vi "LV10_6.vi"() -> ()   [LabVIEW 2014]
uses:
  <vilib>/picture/picture.llb/Draw 8-Bit Pixmap.vi
panel:
  in  "Noise level":dbl(slide) scale=0.0..0.2
  out "Noisy image":picture
  out "Compression ratio":dbl
  in  "Threshold":dbl(slide) scale=0.01..1.0
  out "D3 wavelet transform":picture
  out "Original image":picture
  in  "Stop Button":bool
  out "Reconstructed image":picture
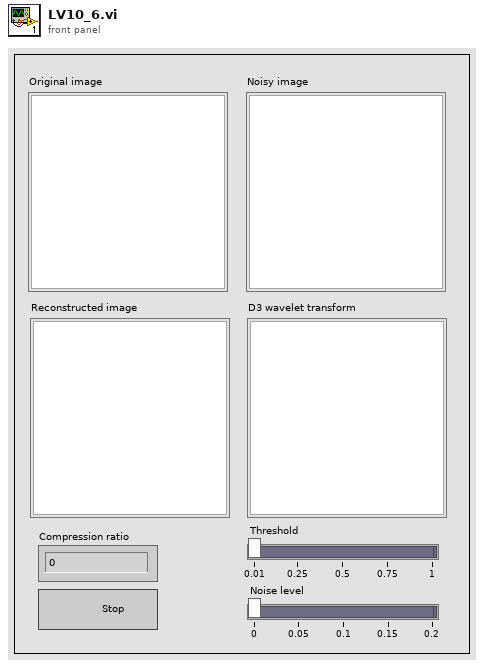
[diagram p1: front panel]
types:
  T1 = typedef "imagedata.ctl" = cluster{"image type":i32, "image depth":i32, "image":u8[], "mask":u8[], "colors":u32[], "Rectangle":cluster{"left":i16, "top":i16, "right":i16, "bottom":i16}}
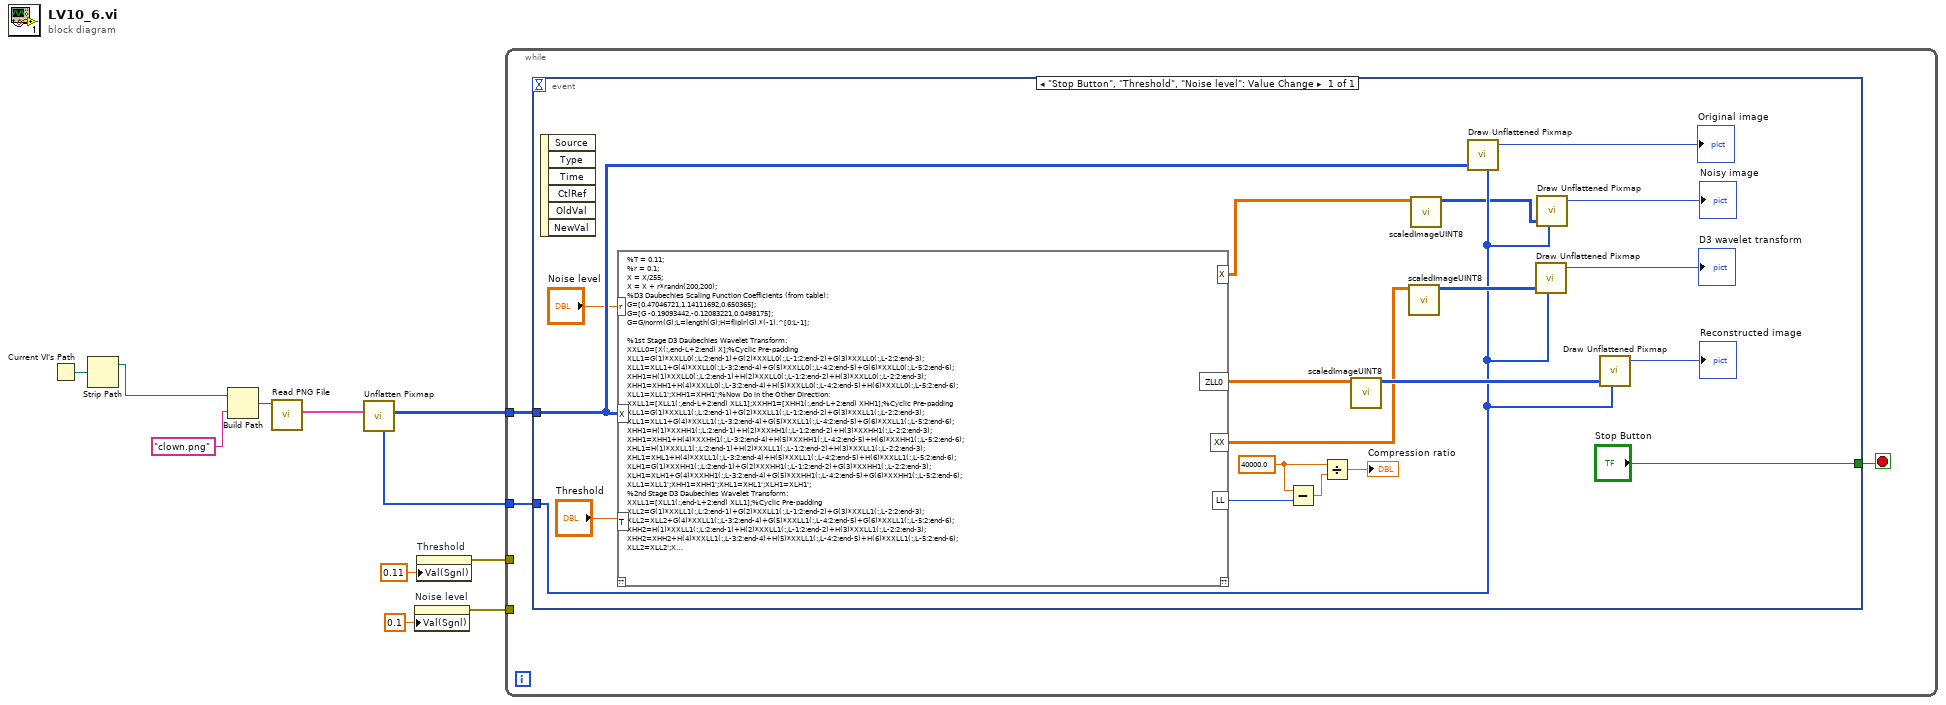
[diagram p0: block diagram]
diagram:
  n1 = Current VI's Path() -> (path=w11:path)
  n2 = Strip Path(path=w11) -> (stripped path=w1:path)  [unwired: 1 out]
  n3 = Build Path(base path=w1, name or relative path="clown.png") -> (appended path=w8:path)
  n4 = call <vilib>:"Read PNG File.vi"("path to PNG file"=w8) -> ("image data"=w7:T1)  [unwired: 8 in, 2 out]
  n5 = call <vilib>:"Unflatten Pixmap.vi"("image data"=w7) -> ("8-bit pixmap"=w9:u8[][], "colors"=w6:u32[])  [unwired: 4 in, 5 out]
  n6 = property on="Noise level" class="Slide (strict)"("Val(Sgnl)"=0.1 ("Value (Signaling)")) -> (error out=w3:errorcluster)  [unwired: 2 in, 1 out]
  n7 = property on="Threshold" class="Slide (strict)"("Val(Sgnl)"=0.11 ("Value (Signaling)")) -> (error out=w5:errorcluster)  [unwired: 2 in, 1 out]
  n8 = while {
    tunnel: w9 -> [w13]
    tunnel: w6 -> [w12]
    tunnel: w5 -> [_]
    tunnel: w3 -> [_]
    stop <- w14 stop-if-true
    n9 = event shown="[0] \"Stop Button\", \"Threshold\", \"Noise level\": Value Change" {
      selector: _ -> [_]
      dyn-events: _ -> [_]
      timeout: _ -> [_]
      tunnel: ["Stop Button"] -> w14
      tunnel: w13 -> [w30]
      tunnel: w12 -> [w17]
      event "Stop Button", "Threshold", "Noise level": Value Change {
        w24 = 40000.0 ("x")
        n10 = event-data() -> ()  [unwired: 1 in, 6 out]
        n11 = mathscript code="%T = 0.11;\n%r = 0.1;\nX = X/255;\nX = X + r*randn(200,200);\n%D3 Daubechies Scaling Function Coefficients (from table):\nG=[0.47046721,1.14111692,0.650365];\nG=[G -0.19093442,-0.12083221,0.0498175];\nG=G/norm(G);L=length(G);H=fliplr(G).*(-1).^[0:L-1];\n\n%1st Stage D3 Daubechies Wavelet Transform:\nXXLL0=[X(:,end-L+2:end) X];%Cyclic Pre-padding\nXLL1=G(1)*XXLL0(:,L:2:end-1)+G(2)*XXLL0(:,L-1:2:end-2)+G(3)*XXLL0(:,L-2:2:end-3);\nXLL1=XLL1+G(4)*XXLL0(:,L-3:2:end-4)+G(5)*XXLL0(:,L-4:2:end-5)+G(6)*XXLL0(:,L-5:2:end-6);\nXHH1=H(1)*XXLL0(:,L:2:end-1)+H(2)*XXLL0(:,L-1:2:end-2)+H(3)*XXLL0(:,L-2:2:end-3);\nXHH1=XHH1+H(4)*XXLL0(:,L-3:2:end-4)+H(5)*XXLL0(:,L-4:2:end-5)+H(6)*XXLL0(:,L-5:2:end-6);\nXLL1=XLL1';XHH1=XHH1';%Now Do in the Other Direction:\nXXLL1=[XLL1(:,end-L+2:end) XLL1];XXHH1=[XHH1(:,end-L+2:end) XHH1];%Cyclic Pre-padding\nXLL1=G(1)*XXLL1(:,L:2:end-1)+G(2)*XXLL1(:,L-1:2:end-2)+G(3)*XXLL1(:,L-2:2:end-3);\nXLL1=XLL1+G(4)*XXLL1(:,L-3:2:end-4)+G(5)*XXLL1(:,L-4:2:end-5)+G(6)*XXLL1(:,L-5:2:end-6);\nXHH1=H(1)*XXHH1(:,L:2:end-1)+H(2)*XXHH1(:,L-1:2:end-2)+H(3)*XXHH1(:,L-2:2:end-3);\nXHH1=XHH1+H(4)*XXHH1(:,L-3:2:end-4)+H(5)*XXHH1(:,L-4:2:end-5)+H(6)*XXHH1(:,L-5:2:end-6);\nXHL1=H(1)*XXLL1(:,L:2:end-1)+H(2)*XXLL1(:,L-1:2:end-2)+H(3)*XXLL1(:,L-2:2:end-3);\nXHL1=XHL1+H(4)*XXLL1(:,L-3:2:end-4)+H(5)*XXLL1(:,L-4:2:end-5)+H(6)*XXLL1(:,L-5:2:end-6);\nXLH1=G(1)*XXHH1(:,L:2:end-1)+G(2)*XXHH1(:,L-1:2:end-2)+G(3)*XXHH1(:,L-2:2:end-3);\nXLH1=XLH1+G(4)*XXHH1(:,L-3:2:end-4)+G(5)*XXHH1(:,L-4:2:end-5)+G(6)*XXHH1(:,L-5:2:end-6);\nXLL1=XLL1';XHH1=XHH1';XHL1=XHL1';XLH1=XLH1';\n%2nd Stage D3 Daubechies Wavelet Transform:\nXXLL1=[XLL1(:,end-L+2:end) XLL1];%Cyclic Pre-padding\nXLL2=G(1)*XXLL1(:,L:2:end-1)+G(2)*XXLL1(:,L-1:2:end-2)+G(3)*XXLL1(:,L-2:2:end-3);\nXLL2=XLL2+G(4)*XXLL1(:,L-3:2:end-4)+G(5)*XXLL1(:,L-4:2:end-5)+G(6)*XXLL1(:,L-5:2:end-6);\nXHH2=H(1)*XXLL1(:,L:2:end-1)+H(2)*XXLL1(:,L-1:2:end-2)+H(3)*XXLL1(:,L-2:2:end-3);\nXHH2=XHH2+H(4)*XXLL1(:,L-3:2:end-4)+H(5)*XXLL1(:,L-4:2:end-5)+H(6)*XXLL1(:,L-5:2:end-6);\nXLL2=XLL2';XHH2=XHH2';%Now Do in the Other Direction:\nXXLL2=[XLL2(:,end-L+2:end) XLL2];XXHH2=[XHH2(:,end-L+2:end) XHH2];%Cyclic Pre-padding\nXLL2=G(1)*XXLL2(:,L:2:end-1)+G(2)*XXLL2(:,L-1:2:end-2)+G(3)*XXLL2(:,L-2:2:end-3);\nXLL2=XLL2+G(4)*XXLL2(:,L-3:2:end-4)+G(5)*XXLL2(:,L-4:2:end-5)+G(6)*XXLL2(:,L-5:2:end-6);\nXHH2=H(1)*XXHH2(:,L:2:end-1)+H(2)*XXHH2(:,L-1:2:end-2)+H(3)*XXHH2(:,L-2:2:end-3);\nXHH2=XHH2+H(4)*XXHH2(:,L-3:2:end-4)+H(5)*XXHH2(:,L-4:2:end-5)+H(6)*XXHH2(:,L-5:2:end-6);\nXHL2=H(1)*XXLL2(:,L:2:end-1)+H(2)*XXLL2(:,L-1:2:end-2)+H(3)*XXLL2(:,L-2:2:end-3);\nXHL2=XHL2+H(4)*XXLL2(:,L-3:2:end-4)+H(5)*XXLL2(:,L-4:2:end-5)+H(6)*XXLL2(:,L-5:2:end-6);\nXLH2=G(1)*XXHH2(:,L:2:end-1)+G(2)*XXHH2(:,L-1:2:end-2)+G(3)*XXHH2(:,L-2:2:end-3);\nXLH2=XLH2+G(4)*XXHH2(:,L-3:2:end-4)+G(5)*XXHH2(:,L-4:2:end-5)+G(6)*XXHH2(:,L-5:2:end-6);\nXLL2=XLL2';XHH2=XHH2';XHL2=XHL2';XLH2=XLH2';\n%3rd Stage D3 Daubechies Wavelet Transform:\nXXLL2=[XLL2(:,end-L+2:end) XLL2];%Cyclic Pre-padding\nXLL3=G(1)*XXLL2(:,L:2:end-1)+G(2)*XXLL2(:,L-1:2:end-2)+G(3)*XXLL2(:,L-2:2:end-3);\nXLL3=XLL3+G(4)*XXLL2(:,L-3:2:end-4)+G(5)*XXLL2(:,L-4:2:end-5)+G(6)*XXLL2(:,L-5:2:end-6);\nXHH3=H(1)*XXLL2(:,L:2:end-1)+H(2)*XXLL2(:,L-1:2:end-2)+H(3)*XXLL2(:,L-2:2:end-3);\nXHH3=XHH3+H(4)*XXLL2(:,L-3:2:end-4)+H(5)*XXLL2(:,L-4:2:end-5)+H(6)*XXLL2(:,L-5:2:end-6);\nXLL3=XLL3';XHH3=XHH3';%Now Do in the Other Direction:\nXXLL3=[XLL3(:,end-L+2:end) XLL3];XXHH3=[XHH3(:,end-L+2:end) XHH3];%Cyclic Pre-padding\nXLL3=G(1)*XXLL3(:,L:2:end-1)+G(2)*XXLL3(:,L-1:2:end-2)+G(3)*XXLL3(:,L-2:2:end-3);\nXLL3=XLL3+G(4)*XXLL3(:,L-3:2:end-4)+G(5)*XXLL3(:,L-4:2:end-5)+G(6)*XXLL3(:,L-5:2:end-6);\nXHH3=H(1)*XXHH3(:,L:2:end-1)+H(2)*XXHH3(:,L-1:2:end-2)+H(3)*XXHH3(:,L-2:2:end-3);\nXHH3=XHH3+H(4)*XXHH3(:,L-3:2:end-4)+H(5)*XXHH3(:,L-4:2:end-5)+H(6)*XXHH3(:,L-5:2:end-6);\nXHL3=H(1)*XXLL3(:,L:2:end-1)+H(2)*XXLL3(:,L-1:2:end-2)+H(3)*XXLL3(:,L-2:2:end-3);\nXHL3=XHL3+H(4)*XXLL3(:,L-3:2:end-4)+H(5)*XXLL3(:,L-4:2:end-5)+H(6)*XXLL3(:,L-5:2:end-6);\nXLH3=G(1)*XXHH3(:,L:2:end-1)+G(2)*XXHH3(:,L-1:2:end-2)+G(3)*XXHH3(:,L-2:2:end-3);\nXLH3=XLH3+G(4)*XXHH3(:,L-3:2:end-4)+G(5)*XXHH3(:,L-4:2:end-5)+G(6)*XXHH3(:,L-5:2:end-6);\nXLL3=XLL3';XHH3=XHH3';XHL3=XHL3';XLH3=XLH3';\n%Wavelet Transform:{XLL3,XLH?,XHL?,XHH?,?=1,2,3}. Display:\n%First, threshold small values of XLH?,XHL?,XHH? to 0.\n%Next 3 lines (and value of T) only change from before.\nXLH1(abs(XLH1)<T)=0;XHL1(abs(XHL1)<T)=0;XHH1(abs(XHH1)<T)=0;\nXLH2(abs(XLH2)<T)=0;XHL2(abs(XHL2)<T)=0;XHH2(abs(XHH2)<T)=0;\nXLH3(abs(XLH3)<T)=0;XHL3(abs(XHL3)<T)=0;XHH3(abs(XHH3)<T)=0;\nXX=[XLL3 XLH3;XHL3 XHH3];XX=[XX XLH2;XHL2 XHH2];\nXX=[XX XLH1;XHL1 XHH1];LL=length(find(abs(XX<1e-10)));\n\n%Inverse Wavelet Transform of {XLL3,XLH?,XHL?,XHH?}\n%3rd Stage Reconstruction:\nZZLL3=[XLL3 XLL3(:,1:3)];ZZLH3=[XLH3 XLH3(:,1:3)];\nZZHL3=[XHL3 XHL3(:,1:3)];ZZHH3=[XHH3 XHH3(:,1:3)];\nK=2*size(XLL3,1);\nA2(:,1:2:K)=G(1)*ZZLL3(:,1:end-3)+G(3)*ZZLL3(:,2:end-2)+G(5)*ZZLL3(:,3:end-1);\nA2(:,2:2:K)=G(2)*ZZLL3(:,2:end-2)+G(4)*ZZLL3(:,3:end-1)+G(6)*ZZLL3(:,4:end);\nA2=A2';AA2=[A2 A2(:,1:3)];%Now Do in the Other Direction:\nA2(:,1:2:K)=G(1)*AA2(:,1:end-3)+G(3)*AA2(:,2:end-2)+G(5)*AA2(:,3:end-1);\nA2(:,2:2:K)=G(2)*AA2(:,2:end-2)+G(4)*AA2(:,3:end-1)+G(6)*AA2(:,4:end);\nB2(:,1:2:K)=G(1)*ZZHL3(:,1:end-3)+G(3)*ZZHL3(:,2:end-2)+G(5)*ZZHL3(:,3:end-1);\nB2(:,2:2:K)=G(2)*ZZHL3(:,2:end-2)+G(4)*ZZHL3(:,3:end-1)+G(6)*ZZHL3(:,4:end);\nB2=B2';BB2=[B2 B2(:,1:3)];%Now Do in the Other Direction:\nB2(:,1:2:K)=H(1)*BB2(:,1:end-3)+H(3)*BB2(:,2:end-2)+H(5)*BB2(:,3:end-1);\nB2(:,2:2:K)=H(2)*BB2(:,2:end-2)+H(4)*BB2(:,3:end-1)+H(6)*BB2(:,4:end);\nC2(:,1:2:K)=H(1)*ZZLH3(:,1:end-3)+H(3)*ZZLH3(:,2:end-2)+H(5)*ZZLH3(:,3:end-1);\nC2(:,2:2:K)=H(2)*ZZLH3(:,2:end-2)+H(4)*ZZLH3(:,3:end-1)+H(6)*ZZLH3(:,4:end);\nC2=C2';CC2=[C2 C2(:,1:3)];%Now Do in the Other Direction:\nC2(:,1:2:K)=G(1)*CC2(:,1:end-3)+G(3)*CC2(:,2:end-2)+G(5)*CC2(:,3:end-1);\nC2(:,2:2:K)=G(2)*CC2(:,2:end-2)+G(4)*CC2(:,3:end-1)+G(6)*CC2(:,4:end);\nD2(:,1:2:K)=H(1)*ZZHH3(:,1:end-3)+H(3)*ZZHH3(:,2:end-2)+H(5)*ZZHH3(:,3:end-1);\nD2(:,2:2:K)=H(2)*ZZHH3(:,2:end-2)+H(4)*ZZHH3(:,3:end-1)+H(6)*ZZHH3(:,4:end);\nD2=D2';DD2=[D2 D2(:,1:3)];%Now Do in the Other Direction:\nD2(:,1:2:K)=H(1)*DD2(:,1:end-3)+H(3)*DD2(:,2:end-2)+H(5)*DD2(:,3:end-1);\nD2(:,2:2:K)=H(2)*DD2(:,2:end-2)+H(4)*DD2(:,3:end-1)+H(6)*DD2(:,4:end);\nZLL2=A2+B2+C2+D2;ZLL2=ZLL2';\n%2nd Stage Reconstruction: Use Computed ZLL2 and Given X??2:\nZZLL2=[ZLL2 ZLL2(:,1:3)];ZZLH2=[XLH2 XLH2(:,1:3)];\nZZHL2=[XHL2 XHL2(:,1:3)];ZZHH2=[XHH2 XHH2(:,1:3)];\nK=2*size(ZLL2,1);\nA1(:,1:2:K)=G(1)*ZZLL2(:,1:end-3)+G(3)*ZZLL2(:,2:end-2)+G(5)*ZZLL2(:,3:end-1);\nA1(:,2:2:K)=G(2)*ZZLL2(:,2:end-2)+G(4)*ZZLL2(:,3:end-1)+G(6)*ZZLL2(:,4:end);\nA1=A1';AA1=[A1 A1(:,1:3)];%Now Do in the Other Direction:\nA1(:,1:2:K)=G(1)*AA1(:,1:end-3)+G(3)*AA1(:,2:end-2)+G(5)*AA1(:,3:end-1);\nA1(:,2:2:K)=G(2)*AA1(:,2:end-2)+G(4)*AA1(:,3:end-1)+G(6)*AA1(:,4:end);\nB1(:,1:2:K)=G(1)*ZZHL2(:,1:end-3)+G(3)*ZZHL2(:,2:end-2)+G(5)*ZZHL2(:,3:end-1);\nB1(:,2:2:K)=G(2)*ZZHL2(:,2:end-2)+G(4)*ZZHL2(:,3:end-1)+G(6)*ZZHL2(:,4:end);\nB1=B1';BB1=[B1 B1(:,1:3)];%Now Do in the Other Direction:\nB1(:,1:2:K)=H(1)*BB1(:,1:end-3)+H(3)*BB1(:,2:end-2)+H(5)*BB1(:,3:end-1);\nB1(:,2:2:K)=H(2)*BB1(:,2:end-2)+H(4)*BB1(:,3:end-1)+H(6)*BB1(:,4:end);\nC1(:,1:2:K)=H(1)*ZZLH2(:,1:end-3)+H(3)*ZZLH2(:,2:end-2)+H(5)*ZZLH2(:,3:end-1);\nC1(:,2:2:K)=H(2)*ZZLH2(:,2:end-2)+H(4)*ZZLH2(:,3:end-1)+H(6)*ZZLH2(:,4:end);\nC1=C1';CC1=[C1 C1(:,1:3)];%Now Do in the Other Direction:\nC1(:,1:2:K)=G(1)*CC1(:,1:end-3)+G(3)*CC1(:,2:end-2)+G(5)*CC1(:,3:end-1);\nC1(:,2:2:K)=G(2)*CC1(:,2:end-2)+G(4)*CC1(:,3:end-1)+G(6)*CC1(:,4:end);\nD1(:,1:2:K)=H(1)*ZZHH2(:,1:end-3)+H(3)*ZZHH2(:,2:end-2)+H(5)*ZZHH2(:,3:end-1);\nD1(:,2:2:K)=H(2)*ZZHH2(:,2:end-2)+H(4)*ZZHH2(:,3:end-1)+H(6)*ZZHH2(:,4:end);\nD1=D1';DD1=[D1 D1(:,1:3)];%Now Do in the Other Direction:\nD1(:,1:2:K)=H(1)*DD1(:,1:end-3)+H(3)*DD1(:,2:end-2)+H(5)*DD1(:,3:end-1);\nD1(:,2:2:K)=H(2)*DD1(:,2:end-2)+H(4)*DD1(:,3:end-1)+H(6)*DD1(:,4:end);\nZLL1=A1+B1+C1+D1;ZLL1=ZLL1';\n%1st Stage Reconstruction: Use Computed ZLL1 and Given X??1:\nZZLL1=[ZLL1 ZLL1(:,1:3)];ZZLH1=[XLH1 XLH1(:,1:3)];\nZZHL1=[XHL1 XHL1(:,1:3)];ZZHH1=[XHH1 XHH1(:,1:3)];\nK=2*size(ZLL1,1);\nA0(:,1:2:K)=G(1)*ZZLL1(:,1:end-3)+G(3)*ZZLL1(:,2:end-2)+G(5)*ZZLL1(:,3:end-1);\nA0(:,2:2:K)=G(2)*ZZLL1(:,2:end-2)+G(4)*ZZLL1(:,3:end-1)+G(6)*ZZLL1(:,4:end);\nA0=A0';AA0=[A0 A0(:,1:3)];%Now Do in the Other Direction:\nA0(:,1:2:K)=G(1)*AA0(:,1:end-3)+G(3)*AA0(:,2:end-2)+G(5)*AA0(:,3:end-1);\nA0(:,2:2:K)=G(2)*AA0(:,2:end-2)+G(4)*AA0(:,3:end-1)+G(6)*AA0(:,4:end);\nB0(:,1:2:K)=G(1)*ZZHL1(:,1:end-3)+G(3)*ZZHL1(:,2:end-2)+G(5)*ZZHL1(:,3:end-1);\nB0(:,2:2:K)=G(2)*ZZHL1(:,2:end-2)+G(4)*ZZHL1(:,3:end-1)+G(6)*ZZHL1(:,4:end);\nB0=B0';BB0=[B0 B0(:,1:3)];%Now Do in the Other Direction:\nB0(:,1:2:K)=H(1)*BB0(:,1:end-3)+H(3)*BB0(:,2:end-2)+H(5)*BB0(:,3:end-1);\nB0(:,2:2:K)=H(2)*BB0(:,2:end-2)+H(4)*BB0(:,3:end-1)+H(6)*BB0(:,4:end);\nC0(:,1:2:K)=H(1)*ZZLH1(:,1:end-3)+H(3)*ZZLH1(:,2:end-2)+H(5)*ZZLH1(:,3:end-1);\nC0(:,2:2:K)=H(2)*ZZLH1(:,2:end-2)+H(4)*ZZLH1(:,3:end-1)+H(6)*ZZLH1(:,4:end);\nC0=C0';CC0=[C0 C0(:,1:3)];%Now Do in the Other Direction:\nC0(:,1:2:K)=G(1)*CC0(:,1:end-3)+G(3)*CC0(:,2:end-2)+G(5)*CC0(:,3:end-1);\nC0(:,2:2:K)=G(2)*CC0(:,2:end-2)+G(4)*CC0(:,3:end-1)+G(6)*CC0(:,4:end);\nD0(:,1:2:K)=H(1)*ZZHH1(:,1:end-3)+H(3)*ZZHH1(:,2:end-2)+H(5)*ZZHH1(:,3:end-1);\nD0(:,2:2:K)=H(2)*ZZHH1(:,2:end-2)+H(4)*ZZHH1(:,3:end-1)+H(6)*ZZHH1(:,4:end);\nD0=D0';DD0=[D0 D0(:,1:3)];%Now Do in the Other Direction:\nD0(:,1:2:K)=H(1)*DD0(:,1:end-3)+H(3)*DD0(:,2:end-2)+H(5)*DD0(:,3:end-1);\nD0(:,2:2:K)=H(2)*DD0(:,2:end-2)+H(4)*DD0(:,3:end-1)+H(6)*DD0(:,4:end);\nZLL0=A0+B0+C0+D0;ZLL0=ZLL0';"("X"=w30, "T"="Threshold", "r"="Noise level") -> ("ZLL0"=w27:dbl[][], "XX"=w25:dbl[][], "LL"=w23:i32, "X"=w18:dbl[][])  [unwired: 1 in, 1 out]
        n12 = Subtract(x=w24, y=w23) -> (x-y=w22:dbl)
        n13 = Divide(x=w24, y=w22) -> (x/y=→"Compression ratio":dbl)
        n14 = call "scaledImageUINT8.vi"("double image"=w27) -> ("uint8 image"=w26:u8[][])  [unwired: 10 in]
        n15 = call "scaledImageUINT8.vi"("double image"=w25) -> ("uint8 image"=w28:u8[][])  [unwired: 10 in]
        n16 = call "scaledImageUINT8.vi"("double image"=w18) -> ("uint8 image"=w16:u8[][])  [unwired: 10 in]
        n17 = call-poly <vilib>:"Draw Unflattened Pixmap.vi"("data"=w30, "color table"=w17) -> ("new picture"=→"Original image":picture)  [unwired: 7 in]
        n18 = call-poly <vilib>:"Draw Unflattened Pixmap.vi"("data"=w28, "color table"=w17) -> ("new picture"=→"D3 wavelet transform":picture)  [unwired: 7 in]
        n19 = call-poly <vilib>:"Draw Unflattened Pixmap.vi"("data"=w16, "color table"=w17) -> ("new picture"=→"Noisy image":picture)  [unwired: 7 in]
        n20 = call-poly <vilib>:"Draw Unflattened Pixmap.vi"("data"=w26, "color table"=w17) -> ("new picture"=→"Reconstructed image":picture)  [unwired: 7 in]
      }
    }
  }
